vi "Verify Non NI Instruments.vi"(5 "instrument types in":string[](array[string])) -> (2 "instrument types out":string[](array[string]))   [LabVIEW 2021, in "Converter.lvlib"]
uses:
  Converter.lvlib
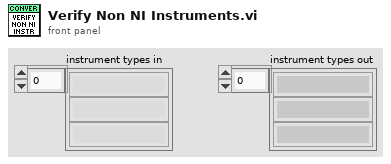
[diagram p1: front panel]
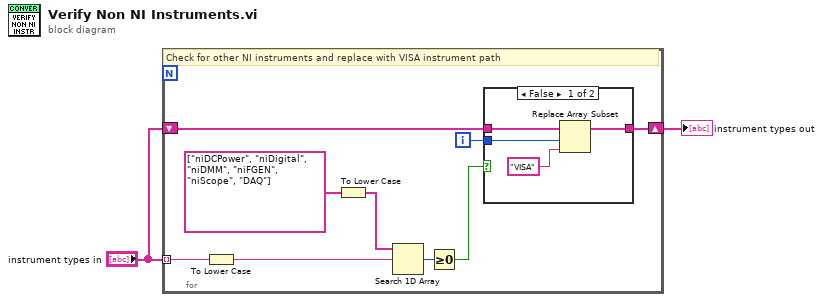
[diagram p0: block diagram]
diagram:
  n1 = for {
    tunnel: "instrument types in" -> [w11] mode=indexing
    shift-right: [w8] -> w1
    shift-left: "instrument types in" -> [w9]
    i -> [w7]
    # "Check for other NI instruments and replace with VISA instrument path"
    n2 = To Lower Case(string=w11) -> (all lower case string=w5:string)
    n3 = To Lower Case(string=string[] ["niDCPower", "niDigital", "niDMM", "niFGEN", "niScope", "DAQ"] ("regular expression")) -> (all lower case string=w3:string[])
    n4 = Search 1D Array(1D array=w3, element=w5) -> (index of element=w10:i32)  [unwired: 1 in]
    n5 = Greater Or Equal To 0?(x=w10) -> (x >= 0?=w6:bool)
    n6 = case shown="False" w6 {
      tunnel: w9 -> [w15 w16]
      tunnel: [w14 w16] -> w8
      tunnel: w7 -> [w13 _]
      frame False {
        n7 = Replace Array Subset(array=w15, new element="VISA" ("new element/subarray"), index=w13) -> (w14:string[])
      }
      frame True {
      }
    }
  }
  "instrument types out" <- w1
